vi "Create Global MetaData Channel - Single Channel - Format.vi"(8 "error in (no error)":errorcluster, 9 "settings":T1, 10 "channel name":string, 11 "instrument addon refnum in":T2=18446744073709551615 format="%.0x") -> (0 "error out":errorcluster, 2 "channel refnum":T2=18446744073709551615 format="%.0x", 3 "instrument addon refnum out":T2=18446744073709551615 format="%.0x")   [LabVIEW 2019, in "Instrument Addon Scripting API.lvlib"]
doc: "Creates a new channel in the Global MetaData Channels section of the specified Instrument Addon Custom Device."
uses:
  Instrument Addon Scripting API.lvlib
  <vilib>/NI VeriStand/Custom Device API/Custom Device Item Ref.ctl
  TypeDefs/Single Channel Format Settings.ctl
  Addon/Addon Shared/Types/MetaData Parameters.ctl
  Addon/Addon Shared/Types/Protocol Data Type.ctl
  Addon/Addon Shared/Types/Metadata Channel Type.ctl
  Addon/Addon Shared/Types/Type Cast Type.ctl
  Addon/Addon Shared/Types/Endian.ctl
  TypeDefs/Channel Properties.ctl
  Addon/Addon Shared/Instrument Addon Shared.lvlib
  <vilib>/NI VeriStand/Custom Device API/Custom Device API.lvlib
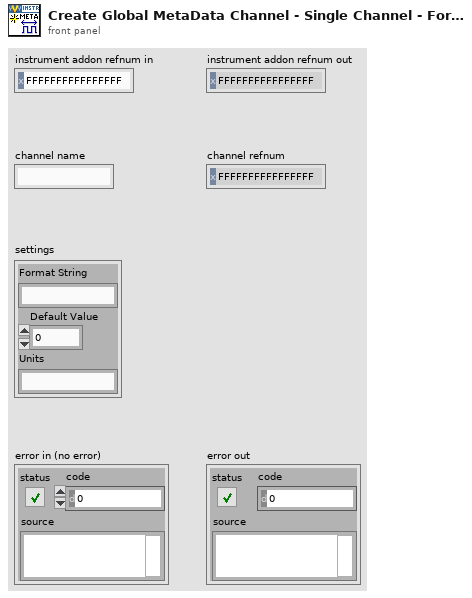
[diagram p1: front panel]
types:
  T1 = typedef "Instrument Addon Scripting API.lvlib/Single Channel Format Settings.ctl" = cluster{"Format String":string, "Default Value":dbl, "Units":string}
  T2 = typedef "Custom Device API.lvlib/Custom Device Item Ref.ctl" = u64
  T3 = typedef "Instrument Addon Scripting API.lvlib/Channel Properties.ctl" = cluster{"Default Value":dbl, "Units":string}
  T4 = typedef "Instrument Addon Shared.lvlib/Metadata Channel Type.ctl" = enum16{"Enumerated List", "Format", "Type Cast"}
  T5 = typedef "Instrument Addon Shared.lvlib/Protocol Data Type.ctl" = enum16{"Single Channel", "Array"}
  T6 = typedef "Instrument Addon Shared.lvlib/MetaData Parameters.ctl" = cluster{"Data Type":T5, "Channel Type":T4, "List":string[], "Format String":string, "Type":T7, "Delimiter":string, "Endian":T8}
  T7 = typedef "Instrument Addon Shared.lvlib/Type Cast Type.ctl" = enum16{"DBL", "SGL", "U64", "U32", "U16", "U8", "I64", "I32", "I16", "I8"}
  T8 = typedef "Instrument Addon Shared.lvlib/Endian.ctl" = enum16{"Native", "Little", "Big"}
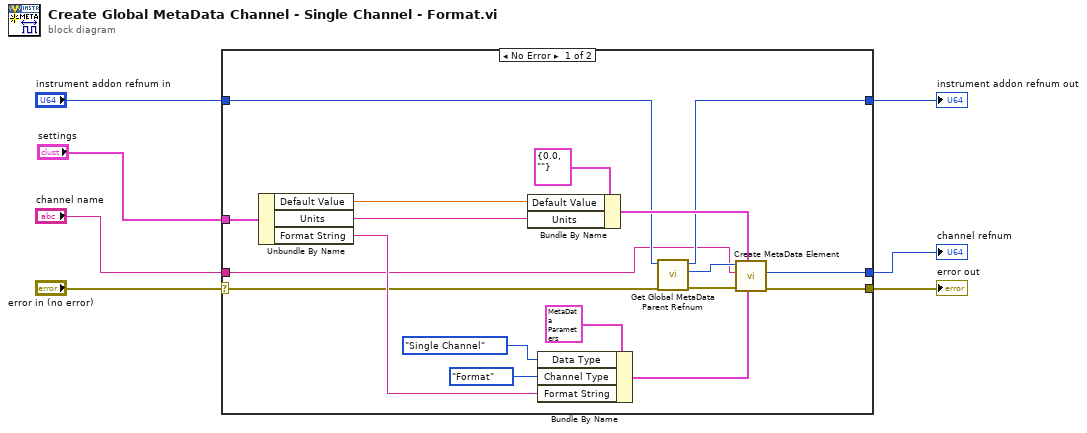
[diagram p0: block diagram]
diagram:
  n1 = case shown="No Error" "error in (no error)" {
    selector: "error in (no error)" -> [w13 w26]
    tunnel: [w25 w26] -> w7
    tunnel: "settings" -> [w24 _]
    tunnel: "instrument addon refnum in" -> [w9 w27]
    tunnel: [w14 _] -> w5
    tunnel: [w10 w27] -> w4
    tunnel: "channel name" -> [w8 _]
    frame No Error {
      n2 = Unbundle By Name(w24) -> ("Default Value"=w18:dbl, "Units"=w17:string, "Format String"=w20:string)
      n3 = Bundle By Name(cluster=T3 {"Default Value"=0.0, "Units"=""}, "Default Value"=w18, "Units"=w17) -> (w15:T3)
      n4 = Bundle By Name(cluster=T6 {"Data Type"=enum."Single Channel", "Channel Type"=enum."Format", "List"=[], "Format String"="%.3g", "Type"=enum."SGL", "Delimiter"="", "Endian"=enum."Native"} ("MetaData Parameters"), "Data Type"=Protocol_Data_Type."Single Channel", "Channel Type"=Metadata_Channel_Type."Format", "Format String"=w20) -> (w19:T6)
      n5 = call "Get Global MetaData Parent Refnum.vi"("error in (no error)"=w13, "instrument addon refnum in"=w9) -> ("error out"=w12:errorcluster, "global metadata section refnum"=w11:T2, "instrument addon refnum out"=w10:T2)  [unwired: 7 in]
      n6 = call "Create MetaData Element.vi"("MetaData Parameters"=w19, "Channel Properties"=w15, "error in (no error)"=w12, "Name"=w8, "Refnum In"=w11) -> ("error out"=w25:errorcluster, "Channel Refnum"=w14:T2)  [unwired: 4 in, 1 out]
    }
    frame Error {
    }
  }
  "instrument addon refnum out" <- w4
  "error out" <- w7
  "channel refnum" <- w5
